vi "GetFirstDeviceID.vi"(3 "error in":errorcluster, 5 "DevInfoList In":refnum<k24>) -> (0 "error out":errorcluster, 1 "Device ID":i32, 2 "DevInfoList Out":refnum<k24>)   [LabVIEW 2009]
uses:
  C:/Samples/LabVIEW/FilterByProductID/LabVIEW 2009/UsbDllWrap.dll
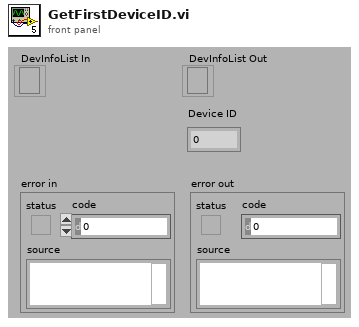
[diagram p1: front panel]
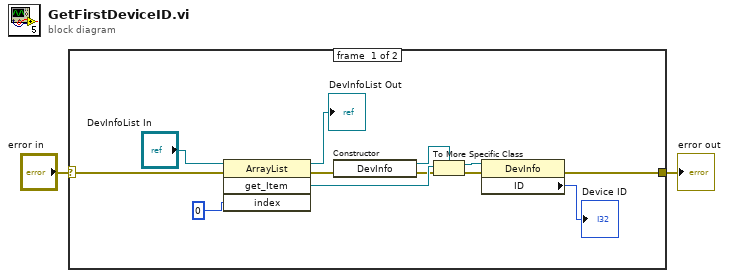
[diagram p0: block diagram]
diagram:
  n1 = case shown="No Error" "error in" {
    selector: "error in" -> [w3 w15]
    tunnel: [w12 w15] -> w2
    frame #0 {
      n2 = invoke class="ArrayList" method="get_Item"(reference="DevInfoList In", error in=w3, "index"=0) -> (reference out=→"DevInfoList Out":refnum<k24>, error out=w14:errorcluster, "get_Item"=w11:refnum<k24>)  [unwired: 1 in, 1 out]
      n3 = constructor class="DevInfo"(error in=w14) -> (reference out=w8:refnum<k24>, error out=w7:errorcluster)  [unwired: 2 in, 1 out]
      n4 = To More Specific Class(target class=w8, reference=w11, error in=w7) -> (specific class reference=w9:refnum<k24>, error out=w10:errorcluster)
      n5 = property class="DevInfo"(reference=w9, error in=w10) -> (error out=w12:errorcluster, "ID"=→"Device ID":i32)  [unwired: 1 out]
    }
    frame #1 {
    }
  }
  "error out" <- w2
